vi "Create Element.vi"(8 "Attributes":refnum<class "Attribute.lvclass">[](array[class]), 9 "elements":string, 10 "uid":string, 11 "class":string) -> (3 "Element":refnum<class "Element.lvclass">)   [LabVIEW 2026, in "VILab.lvlib" / "Element.lvclass"]
uses:
  Element.lvclass
  Attribute/Attribute.lvclass
  Element.lvclass/Element.ctl
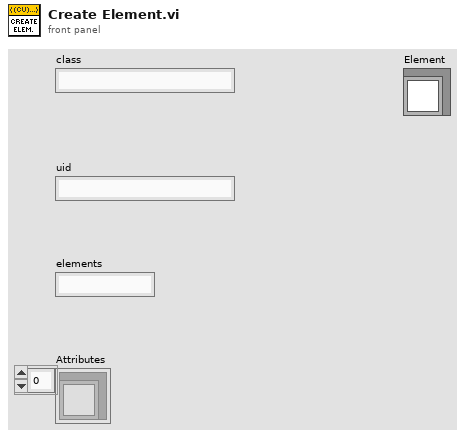
[diagram p1: front panel]
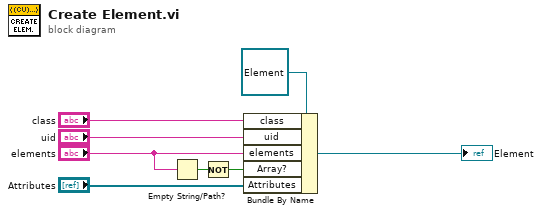
[diagram p0: block diagram]
diagram:
  n1 = Empty String/Path?(string/path="elements") -> (empty?=w2:bool)
  n2 = Not(x=w2) -> (.not. x?=w1:bool)
  n3 = Bundle By Name(cluster=refnum<class "Element.lvclass"> refnum ("VILab.lvlib:Element.lvclass"), "class"="class", "uid"="uid", "elements"="elements", "Array?"=w1, "Attributes"="Attributes") -> (→"Element":refnum<class "Element.lvclass">)
